vi "USB2XXX_FastLINTest.vi"() -> ()   [LabVIEW 2019]
panel:
  out "return type":i32
  out "pData out":u8[](array[numeric])
  in  "Flags":u8
  in  "pData":u8[](array[numeric])=array[4097 elements]
  in  "Len":u32
  in  "Power State":u8(ring)=2 items=["0V", "12V", "5V"]
  in  "BaudRate":u32=20000
  in  "Channel Index":u8(ring) items=["LIN1", "LIN2"]
  in  "Device Index":i32(ring) items=["0", "1", "2", "3", "4", "5"]
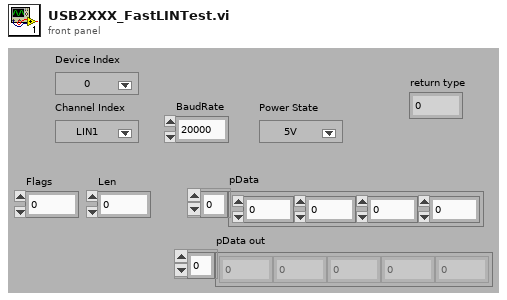
[diagram p1: front panel]
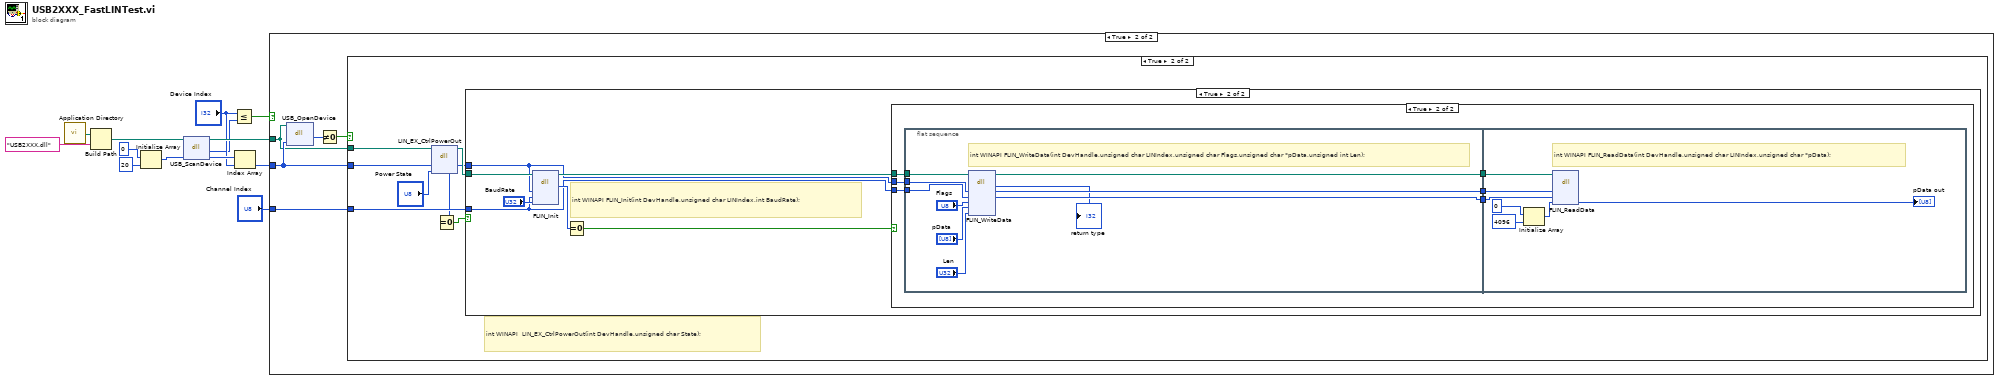
[diagram p0: block diagram]
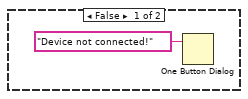
[diagram p2: hidden frame]
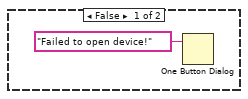
[diagram p3: hidden frame]
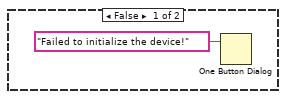
[diagram p5: hidden frame]
diagram:
  n1 = call <vilib>:"Application Directory.vi"() -> ("Application Directory"=w6:path)
  n2 = Build Path(base path=w6, name or relative path="USB2XXX.dll") -> (appended path=w5:path)
  n3 = Initialize Array(0, 20 ("dimension size")) -> (w10:i32[])
  n4 = dll-call lib="E:/OtherWork/STM32/USB2XXX_Example/examples/Labview/PublicFiles/USB2XXX.dll" fn="USB_ScanDevice"(path in=w5, "pDevNum"=w10) -> (path out=w8:path, "return type"=w2:i32, "pDevNum"=w13:i32[])  [unwired: 2 in, 1 out]
  n5 = Less Or Equal?(x="Device Index", y=w2) -> (x <= y?=w4:bool)
  n6 = Index Array(array=w13, index="Device Index") -> (element=w9:i32)
  n7 = case shown="True" w4 {
    tunnel: w9 -> [_ w17]
    tunnel: w8 -> [_ w16]
    tunnel: "Channel Index" -> [_ w15]
    frame False {
      n8 = One Button Dialog(message="Device not connected!") -> ()  [unwired: 1 in, 1 out]
    }
    frame True {
      n9 = dll-call lib="E:/OtherWork/STM32/USB2XXX_Example/examples/Labview/PublicFiles/USB2XXX.dll" fn="USB_OpenDevice"(path in=w16, "DevIndex"=w17) -> ("return type"=w19:u8)  [unwired: 3 in, 2 out]
      n10 = Not Equal To 0?(x=w19) -> (x != 0?=w18:bool)
      n11 = case shown="True" w18 {
        tunnel: w17 -> [_ w25]
        tunnel: w16 -> [_ w27]
        tunnel: w15 -> [_ w28]
        frame False {
          n12 = One Button Dialog(message="Failed to open device!") -> ()  [unwired: 1 in, 1 out]
        }
        frame True {
          # "int WINAPI  LIN_EX_CtrlPowerOut(int DevHandle,unsigned char State);"
          n13 = dll-call lib="E:/Projects/USB2XXX/trunk/USB2XXX/USB2XXX/vs2010/Release/USB2XXX.*" fn="LIN_EX_CtrlPowerOut"(path in=w27, "DevHandle"=w25, "State"="Power State") -> (path out=w26:path, "return type"=w22:i32, "DevHandle"=w24:i32)  [unwired: 3 in, 1 out]
          n14 = Equal To 0?(x=w22) -> (x = 0?=w21:bool)
          n15 = case shown="True" w21 {
            tunnel: w26 -> [_ w34]
            tunnel: w28 -> [_ w29]
            tunnel: w24 -> [_ w31]
            frame False {
            }
            frame True {
              # "int WINAPI FLIN_Init(int DevHandle,unsigned char LINIndex,int BaudRate);"
              n16 = dll-call lib="E:/Projects/USB2XXX/trunk/USB2XXX/USB2XXX/vs2010/Release/USB2XXX.*" fn="FLIN_Init"(path in=w34, "DevHandle"=w31, "LINIndex"=w29, "BaudRate"="BaudRate") -> (path out=w33:path, "return type"=w32:i32)  [unwired: 5 in, 1 out]
              n17 = Equal To 0?(x=w32) -> (x = 0?=w35:bool)
              n18 = case shown="True" w35 {
                tunnel: w29 -> [_ w40]
                tunnel: w31 -> [_ w41]
                tunnel: w33 -> [_ w42]
                frame False {
                  n19 = One Button Dialog(message="Failed to initialize the device!") -> ()  [unwired: 1 in, 1 out]
                }
                frame True {
                  n20 = flat-sequence {
                    tunnel: w42 -> [w49]
                    tunnel: w41 -> [w47]
                    tunnel: w40 -> [w48]
                    tunnel: [w45] -> w39
                    tunnel: [w46] -> w38
                    tunnel: [w44] -> w37
                    tunnel: w39 -> [w58]
                    tunnel: w38 -> [w57]
                    tunnel: w37 -> [w56]
                    frame #0 {
                      # "int WINAPI FLIN_WriteData(int DevHandle,unsigned char LINIndex,unsigned char Flags,unsigned char *pData,unsigned int Len);"
                      n21 = dll-call lib="E:/Projects/USB2XXX/trunk/USB2XXX/USB2XXX/vs2010/Release/USB2XXX.*" fn="FLIN_WriteData"(path in=w49, "DevHandle"=w47, "LINIndex"=w48, "Flags"="Flags", "pData"="pData", "Len"="Len") -> (path out=w44:path, "return type"=→"return type":i32, "DevHandle"=w45:i32, "LINIndex"=w46:u8)  [unwired: 5 in, 1 out]
                    }
                    frame #1 {
                      # "int WINAPI FLIN_ReadData(int DevHandle,unsigned char LINIndex,unsigned char *pData);"
                      n22 = Initialize Array(u8 0 ("element"), 4096 ("dimension size")) -> (w53:u8[])
                      n23 = dll-call lib="E:/Projects/USB2XXX/trunk/USB2XXX/USB2XXX/vs2010/Release/USB2XXX.*" fn="FLIN_ReadData"(path in=w56, "DevHandle"=w58, "LINIndex"=w57, "pData"=w53) -> ("pData"=→"pData out":u8[])  [unwired: 5 in, 2 out]
                    }
                  }
                }
              }
            }
          }
        }
      }
    }
  }
